vi "Valve Button Mapping Global.vi"(8 "Action":T2, 10 "Valve Buttons":refnum<vi>[](array[refnum]), 11 "Valves":T1[](array[typedef])=[enum."NV-1", enum."NV-2", enum."OV-2", enum."OV-4", enum."OV-3", enum."OV-2", enum."NV-2"]) -> (2 "Buttons":refnum<vi>[](array[refnum]), 3 "Valves":T1[](array[typedef]))   [LabVIEW 2015]
uses:
  Valve Button Mapping Global Action.ctl
  Valve Name Enum.ctl
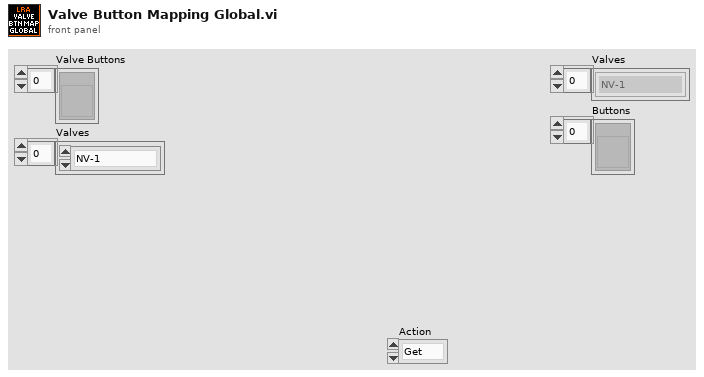
[diagram p1: front panel]
types:
  T1 = typedef "Valve Name Enum.ctl" = enum16{"NV-1", "NV-2", "OV-2", "OV-3", "OV-4", "WV-2"}
  T2 = typedef "Valve Button Mapping Global Action.ctl" = enum16{"Get", "Set"}
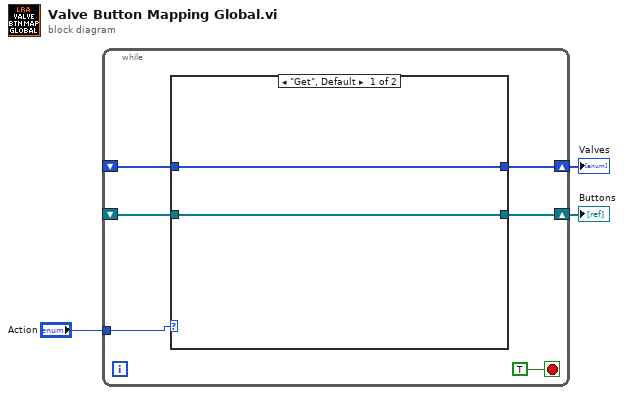
[diagram p0: block diagram]
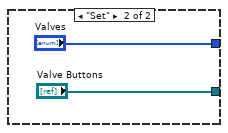
[diagram p2: hidden frame]
diagram:
  n1 = while {
    tunnel: "Action" -> [w8]
    shift-right: [w7] -> w2
    shift-left: _ -> [w5]
    shift-right: [w6] -> w1
    shift-left: _ -> [w4]
    stop <- TRUE stop-if-true
    n2 = case shown="\"Get\", Default" w8 {
      tunnel: [w11 "Valves"] -> w7
      tunnel: [w10 "Valve Buttons"] -> w6
      tunnel: w5 -> [w11 _]
      tunnel: w4 -> [w10 _]
      frame "Get", Default {
      }
      frame "Set" {
      }
    }
  }
  "Valves" <- w2
  "Buttons" <- w1
